vi "Create measurement file.vi"(0 "Global comment":string, 1 "Subfolder":path, 2 "Operator":string, 5 "Row":T2={"Start"=0.0, "Start Caption"="Start [T]", "End"=0.0, "End Caption"="End [T]", "Sweep"=0.0, "Sweep caption"="Rate [mT/s]", "Constant"=0.0, "Constant caption"="Freq [GHz]", "Mod_F [kHz]"=0.0, "Mod_A [G]"=0.0, "Tau [ms]"=0.0, "Positioners [mm|°]"=[], "Tmp [K]"=50.0, "Wait [min]"=0.0, "Carousel"=-1, "Comment"="", "Auto-mod"=TRUE, "Execute"=FALSE} {"Carousel" items=["0", "1", "2", "3", "4", "5", "6"]; "Positioners [mm|°]" min=-1.0 max=330.0; "Tau [ms]" min=0.002 max=10000.0; "Wait [min]" min=0.0 max=3000.0; "Tmp [K]" min=0.0 max=350.0; "Mod_A [G]" min=0.0 max=100.0; "Mod_F [kHz]" min=0.1 max=150.0}, 7 "Sample name":string, 9 "Sample holder":T1, 11 "error in (no error)":errorcluster, 12 "Line index":i32, 13 "Create folder with date":bool) -> (4 "Data file ref out":refnum<file>, 8 "Folder path":path, 15 "error out":errorcluster)   [LabVIEW 2022 SP3]
uses:
  <vilib>/Utility/sysdir.llb/System Directory Type.ctl
  Datatypes/script polymorh line.ctl
  Datatypes/SampleHolders.ctl
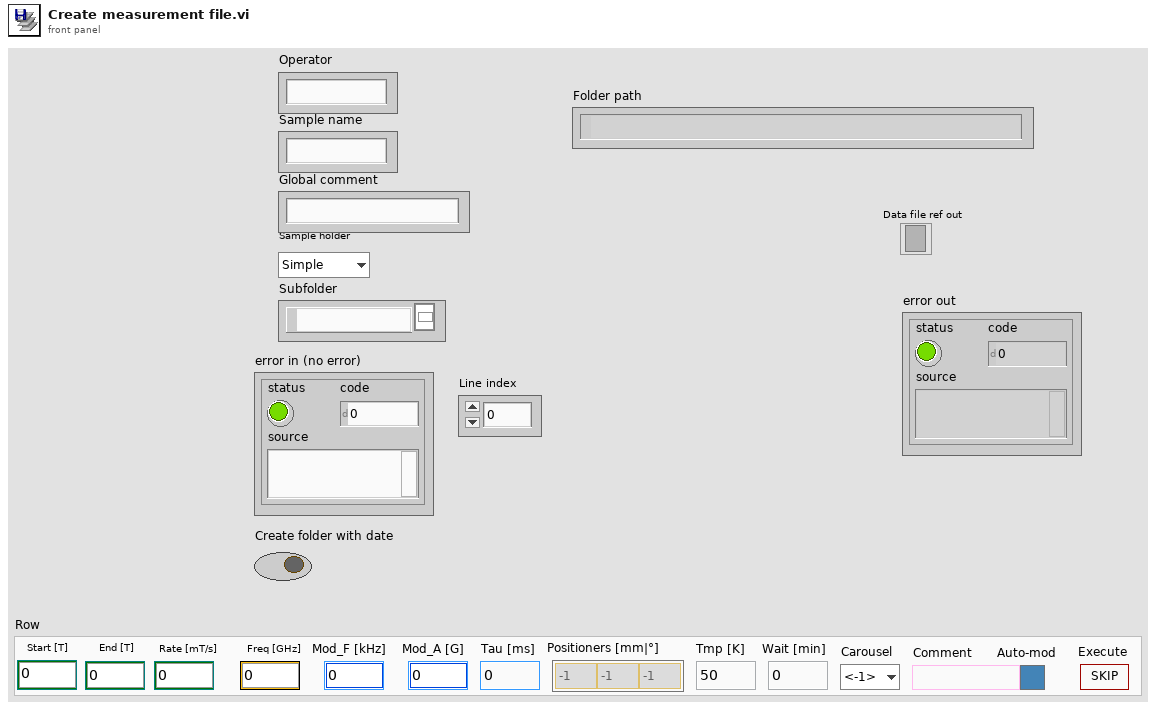
[diagram p1: front panel]
types:
  T1 = typedef "SampleHolders.ctl" = enum16{"Simple", "Carousel", "Chip", "Rotator", "Liquid"}
  T2 = typedef "script polymorh line.ctl" = cluster{"Start":dbl, "Start Caption":string, "End":dbl, "End Caption":string, "Sweep":dbl, "Sweep caption":string, "Constant":dbl, "Constant caption":string, "Mod_F [kHz]":dbl, "Mod_A [G]":dbl, "Tau [ms]":dbl, "Positioners [mm|°]":dbl[], "Tmp [K]":dbl, "Wait [min]":dbl, "Carousel":i8, "Comment":string, "Auto-mod":bool, "Execute":bool}
  T3 = typedef "System Directory Type.ctl" = i32
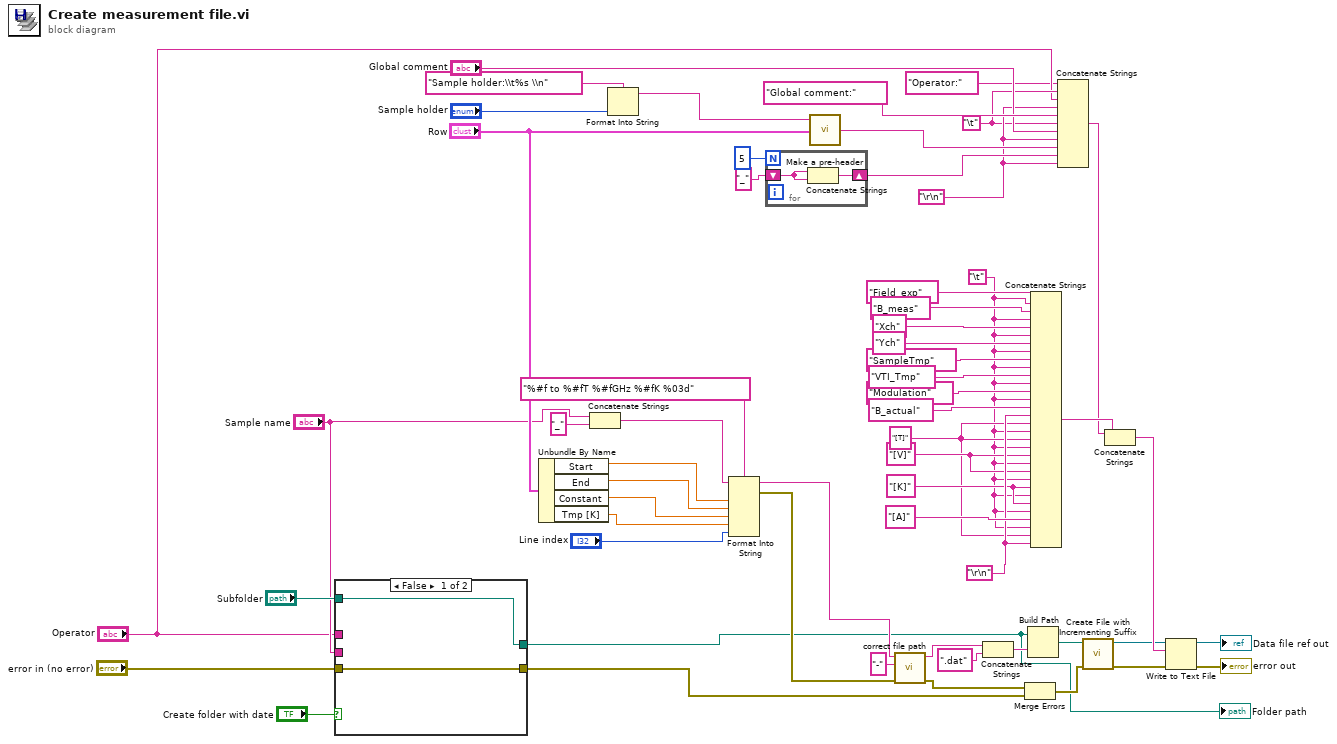
[diagram p0: block diagram]
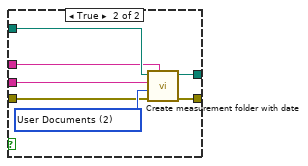
[diagram p2: hidden frame]
diagram:
  w9 = "\t"
  w16 = "\r\n"
  w14 = "[K]"
  w15 = "[V]"
  w2 = "[T]"
  w1 = "\t"
  w10 = "\r\n" ("string")
  n1 = case shown="False" "Create folder with date" {
    tunnel: "Subfolder" -> [w60 w67]
    tunnel: [w60 w66] -> w31
    tunnel: [w59 w65] -> w30
    tunnel: "Sample name" -> [_ w63]
    tunnel: "error in (no error)" -> [w59 w62]
    tunnel: "Operator" -> [_ w61]
    frame False {
    }
    frame True {
      w64 = T3 2 items=["User Home"=0, "User Desktop"=1, "User Documents"=2, "User Application Data"=3, "User Preferences"=4, "User Temporary"=5, "Public Documents"=6, "Public Application Data"=7, "Public Preferences"=8, "Public Cache"=13, "System Core Libraries"=9, "System Installed Libraries"=10, "Application Files"=11, "Boot Volume Root"=12] ("system directory type")
      n2 = call "Create measurement folder with date.vi"("Operator"=w61, "error in (no error)"=w62, "system directory type"=w64, "Sample name"=w63, "Subfolder"=w67) -> ("error out"=w65:errorcluster, "dup path"=w66:path)  [unwired: 5 in]
    }
  }
  "Folder path" <- w31
  n3 = Unbundle By Name("Row") -> ("Start"=w54:dbl, "End"=w53:dbl, "Constant"=w52:dbl, "Tmp [K]"=w6:dbl)
  n4 = Concatenate Strings("Sample name", "_" ("string")) -> (w46:string)
  n5 = Format Into String(format string="Sample holder:\\t%s \\n", "Sample holder") -> (resulting string=w28:string)  [unwired: 2 in, 1 out]
  n6 = Format Into String(format string="%#f to %#fT %#fGHz %#fK %03d", initial string=w46, w54, w53, w52, w6, "Line index") -> (resulting string=w41:string, error out=w33:errorcluster)  [unwired: 1 in]
  n7 = for {
    N: 5 -> [_]
    shift-right: [w69] -> w26
    shift-left: "_" -> [w68]
    n8 = Concatenate Strings(w68, w68) -> (w69:string)
  }
  n9 = call "Make a pre-header.vi"("Row"="Row", "Add to heder comment"=w28) -> ("Pre-header string"=w58:string)  [unwired: 1 in]
  n10 = call "correct file path.vi"("error in (no error)"=w33, "replacement (-)"="-" ("replacement"), "input path"=w41) -> ("error out"=w37:errorcluster, "corrected path"=w42:string)  [unwired: 7 in]
  n11 = Concatenate Strings(w42, ".dat" ("string")) -> (w40:string)
  n12 = Merge Errors(w37, w30) -> (w34:errorcluster)
  n13 = Build Path(base path=w31, name or relative path=w40) -> (appended path=w38:path)
  n14 = Concatenate Strings("Field_exp", w1, "B_meas" ("string"), w1, "Xch", w1, "Ych", w1, "SampleTmp", w1, "VTI_Tmp", w1, "Modulation", w1, "B_actual" ("string"), w16, w2, w1, w2, w1, w15, w1, w15, w1, w14, w1, w14, w1, "[A]", w1, w2, w16) -> (w45:string)
  n15 = Concatenate Strings("Operator:" ("string"), w9, "Operator", w10, "Global comment:" ("string"), w9, "Global comment", w10, w58, w26, w10) -> (w44:string)
  n16 = call <vilib>:"Create File with Incrementing Suffix.vi"("error in (no error)"=w34, "file path"=w38) -> ("error out"=w35:errorcluster, "refnum out"=w36:refnum<file>)  [unwired: 7 in, 1 out]
  n17 = Concatenate Strings(w44, w45) -> (w43:string)
  n18 = Write to Text File(file (use dialog)=w36, text=w43, error in=w35) -> (refnum out=→"Data file ref out":refnum<file>, error out=→"error out":errorcluster)  [unwired: 1 in, 1 out]
